vi "Fill Lists from DB (1st Pass).vi"(4 "error in":errorcluster, 7 "RefNumArray":refnum<vi>[](array[refnum])) -> (0 "error out":errorcluster)   [LabVIEW 2015]
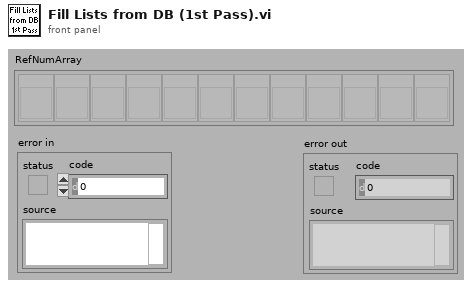
[diagram p1: front panel]
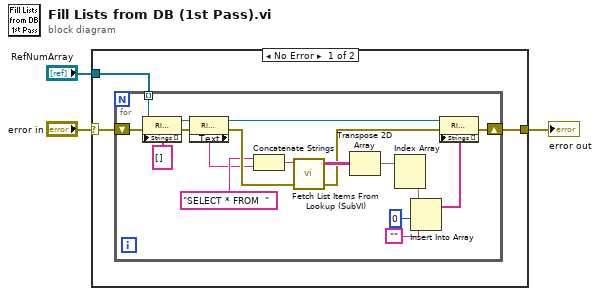
[diagram p0: block diagram]
diagram:
  n1 = case shown="No Error" "error in" {
    selector: "error in" -> [w6 w25]
    tunnel: [w5 w25] -> w2
    tunnel: "RefNumArray" -> [w4 _]
    frame No Error {
      n2 = for {
        tunnel: w4 -> [w14] mode=indexing
        shift-right: [w24] -> w5
        shift-left: w6 -> [w12]
        n3 = property class="Ring (strict)"(reference=w14, error in=w12, "Strings []"=string[] []) -> (reference out=w13:refnum<vi>, error out=w11:errorcluster)
        n4 = property class="Ring (strict)"(reference=w13, error in=w11) -> (reference out=w22:refnum<vi>, error out=w23:errorcluster, "Label.Text"=w8:string)
        n5 = Concatenate Strings("SELECT * FROM  " ("string"), w8) -> (w7:string)
        n6 = call "Fetch List Items From Lookup (SubVI).vi"("error IN"=w23, "Query"=w7) -> ("error OUT"=w20:errorcluster, "recordset data"=w21:string[][])  [unwired: 2 out]
        n7 = Transpose 2D Array(2D array=w21) -> (transposed array=w19:string[][])
        n8 = Index Array(array=w19) -> (element=w16:string[])  [unwired: 2 in]
        n9 = Insert Into Array(array=w16, index=0, new element="" ("new element/subarray")) -> (w15:string[])
        n10 = property class="Ring (strict)"(reference=w22, error in=w20, "Strings []"=w15) -> (error out=w24:errorcluster)  [unwired: 1 out]
      }
    }
    frame Error {
    }
  }
  "error out" <- w2
